vi "CheckShotSuccess.vi"(6 "Vertical Edges":T2(array[cluster]) {"Point2 (Real-World)"."Y" format="%.2f"; "Point2 (Real-World)"."X" format="%.2f"; "Point1 (Real-World)"."Y" format="%.2f"; "Point1 (Real-World)"."X" format="%.2f"; "Point2 (Pixels)"."Y" format="%.2f"; "Point2 (Pixels)"."X" format="%.2f"; "Point1 (Pixels)"."Y" format="%.2f"; "Point1 (Pixels)"."X" format="%.2f"}, 7 "Pixel/mm":dbl format="%#_13g", 8 "error in":errorcluster, 9 "File Path":path, 10 "CameraSettings":T4={"Brightness"=0, "Contrast"=0.0, "Threshold"=50.0}, 11 "Session In":T5) -> (0 "error out":errorcluster, 1 "Image":T1(plugin-control), 2 "Success?":bool, 3 "Session Out":T5, 4 "X distance Out":sgl, 5 "XYPuck":cluster{sgl, sgl})   [LabVIEW 2017]
uses:
  <vilib>/userdefined/High Color/IMAQdx.ctl
panel:
  in  "HomeXY(pixels)":cluster{dbl, dbl}
  out "Vertical Edges[0].Point1 (Pixels).X":sgl
  out "Circles[0].Position.X":sgl
  out "Puck":T3(array[cluster]) {"Position"."Y" format="%.2f"; "Position"."X" format="%.2f"}
  out "Number of Pucks Found":i32
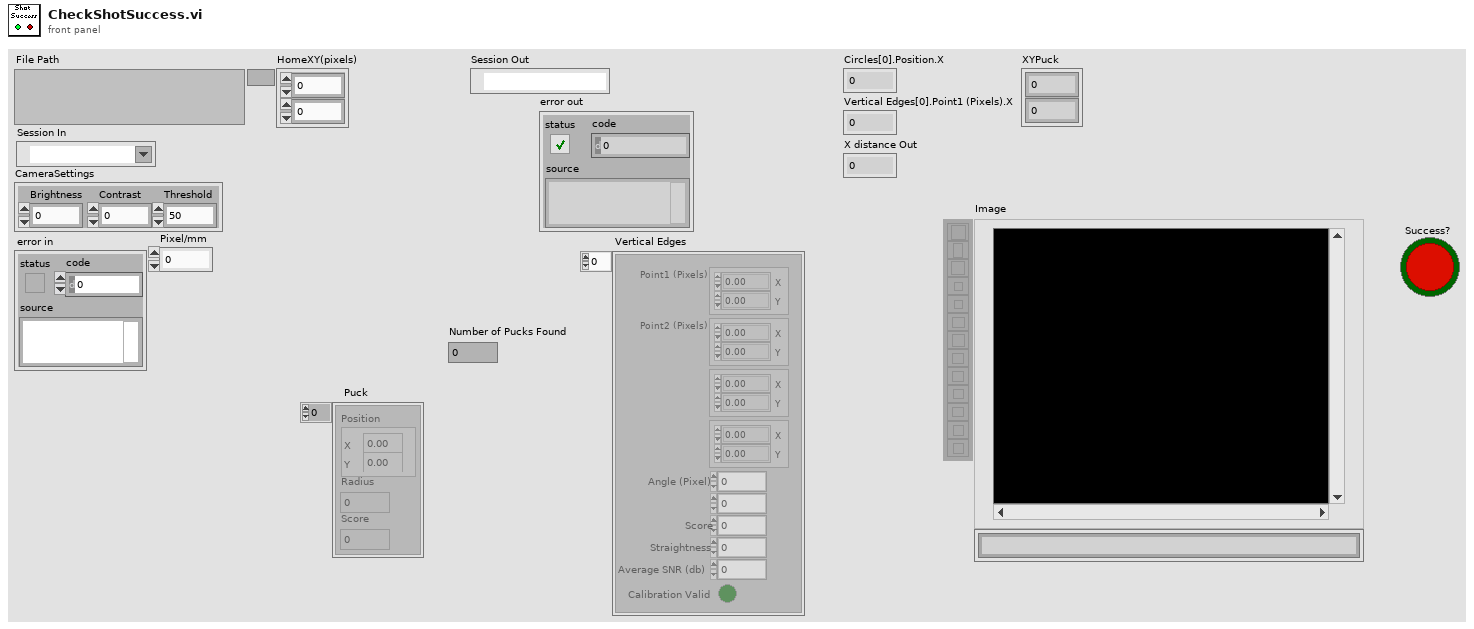
[diagram p1: front panel]
types:
  T1 = typedef "IMAQ Image.ctl" = refnum<image>
  T2 = cluster{"Point1 (Pixels)":cluster{"X":sgl, "Y":sgl}, "Point2 (Pixels)":cluster{"X":sgl, "Y":sgl}, "Point1 (Real-World)":cluster{"X":sgl, "Y":sgl}, "Point2 (Real-World)":cluster{"X":sgl, "Y":sgl}, "Angle (Pixel)":dbl, "Angle (Real-World)":dbl, "Score":dbl, "Straightness":dbl, "Average SNR (db)":dbl, "Calibration Valid":bool}[]
  T3 = cluster{"Position":cluster{"X":sgl, "Y":sgl}, "Radius":dbl, "Score":dbl}[]
  T4 = cluster{"Brightness":i64, "Contrast":dbl, "Threshold":sgl}
  T5 = typedef "IMAQdx.ctl" = refnum<k21>
  T6 = cluster{"Circles[0]":cluster{"Position":cluster{"X":sgl, "Y":sgl}, "Radius":dbl, "Score":dbl}, "Circles[1]":cluster{"Position":cluster{"X":sgl, "Y":sgl}, "Radius":dbl, "Score":dbl}, "Circles[2]":cluster{"Position":cluster{"X":sgl, "Y":sgl}, "Radius":dbl, "Score":dbl}, "Circles[3]":cluster{"Position":cluster{"X":sgl, "Y":sgl}, "Radius":dbl, "Score":dbl}, "Circles[4]":cluster{"Position":cluster{"X":sgl, "Y":sgl}, "Radius":dbl, "Score":dbl}, "Circles[5]":cluster{"Position":cluster{"X":sgl, "Y":sgl}, "Radius":dbl, "Score":dbl}, "Circles[6]":cluster{"Position":cluster{"X":sgl, "Y":sgl}, "Radius":dbl, "Score":dbl}, "Circles[7]":cluster{"Position":cluster{"X":sgl, "Y":sgl}, "Radius":dbl, "Score":dbl}, "Circles[8]":cluster{"Position":cluster{"X":sgl, "Y":sgl}, "Radius":dbl, "Score":dbl}}
  T7 = cluster{"Vertical Edges[0]":cluster{"Point1 (Pixels)":cluster{"X":sgl, "Y":sgl}, "Point2 (Pixels)":cluster{"X":sgl, "Y":sgl}, "Point1 (Real-World)":cluster{"X":sgl, "Y":sgl}, "Point2 (Real-World)":cluster{"X":sgl, "Y":sgl}, "Angle (Pixel)":dbl, "Angle (Real-World)":dbl, "Score":dbl, "Straightness":dbl, "Average SNR (db)":dbl, "Calibration Valid":bool}, "Vertical Edges[1]":cluster{"Point1 (Pixels)":cluster{"X":sgl, "Y":sgl}, "Point2 (Pixels)":cluster{"X":sgl, "Y":sgl}, "Point1 (Real-World)":cluster{"X":sgl, "Y":sgl}, "Point2 (Real-World)":cluster{"X":sgl, "Y":sgl}, "Angle (Pixel)":dbl, "Angle (Real-World)":dbl, "Score":dbl, "Straightness":dbl, "Average SNR (db)":dbl, "Calibration Valid":bool}, "Vertical Edges[2]":cluster{"Point1 (Pixels)":cluster{"X":sgl, "Y":sgl}, "Point2 (Pixels)":cluster{"X":sgl, "Y":sgl}, "Point1 (Real-World)":cluster{"X":sgl, "Y":sgl}, "Point2 (Real-World)":cluster{"X":sgl, "Y":sgl}, "Angle (Pixel)":dbl, "Angle (Real-World)":dbl, "Score":dbl, "Straightness":dbl, "Average SNR (db)":dbl, "Calibration Valid":bool}, "Vertical Edges[3]":cluster{"Point1 (Pixels)":cluster{"X":sgl, "Y":sgl}, "Point2 (Pixels)":cluster{"X":sgl, "Y":sgl}, "Point1 (Real-World)":cluster{"X":sgl, "Y":sgl}, "Point2 (Real-World)":cluster{"X":sgl, "Y":sgl}, "Angle (Pixel)":dbl, "Angle (Real-World)":dbl, "Score":dbl, "Straightness":dbl, "Average SNR (db)":dbl, "Calibration Valid":bool}, "Vertical Edges[4]":cluster{"Point1 (Pixels)":cluster{"X":sgl, "Y":sgl}, "Point2 (Pixels)":cluster{"X":sgl, "Y":sgl}, "Point1 (Real-World)":cluster{"X":sgl, "Y":sgl}, "Point2 (Real-World)":cluster{"X":sgl, "Y":sgl}, "Angle (Pixel)":dbl, "Angle (Real-World)":dbl, "Score":dbl, "Straightness":dbl, "Average SNR (db)":dbl, "Calibration Valid":bool}, "Vertical Edges[5]":cluster{"Point1 (Pixels)":cluster{"X":sgl, "Y":sgl}, "Point2 (Pixels)":cluster{"X":sgl, "Y":sgl}, "Point1 (Real-World)":cluster{"X":sgl, "Y":sgl}, "Point2 (Real-World)":cluster{"X":sgl, "Y":sgl}, "Angle (Pixel)":dbl, "Angle (Real-World)":dbl, "Score":dbl, "Straightness":dbl, "Average SNR (db)":dbl, "Calibration Valid":bool}, "Vertical Edges[6]":cluster{"Point1 (Pixels)":cluster{"X":sgl, "Y":sgl}, "Point2 (Pixels)":cluster{"X":sgl, "Y":sgl}, "Point1 (Real-World)":cluster{"X":sgl, "Y":sgl}, "Point2 (Real-World)":cluster{"X":sgl, "Y":sgl}, "Angle (Pixel)":dbl, "Angle (Real-World)":dbl, "Score":dbl, "Straightness":dbl, "Average SNR (db)":dbl, "Calibration Valid":bool}, "Vertical Edges[7]":cluster{"Point1 (Pixels)":cluster{"X":sgl, "Y":sgl}, "Point2 (Pixels)":cluster{"X":sgl, "Y":sgl}, "Point1 (Real-World)":cluster{"X":sgl, "Y":sgl}, "Point2 (Real-World)":cluster{"X":sgl, "Y":sgl}, "Angle (Pixel)":dbl, "Angle (Real-World)":dbl, "Score":dbl, "Straightness":dbl, "Average SNR (db)":dbl, "Calibration Valid":bool}, "Vertical Edges[8]":cluster{"Point1 (Pixels)":cluster{"X":sgl, "Y":sgl}, "Point2 (Pixels)":cluster{"X":sgl, "Y":sgl}, "Point1 (Real-World)":cluster{"X":sgl, "Y":sgl}, "Point2 (Real-World)":cluster{"X":sgl, "Y":sgl}, "Angle (Pixel)":dbl, "Angle (Real-World)":dbl, "Score":dbl, "Straightness":dbl, "Average SNR (db)":dbl, "Calibration Valid":bool}}
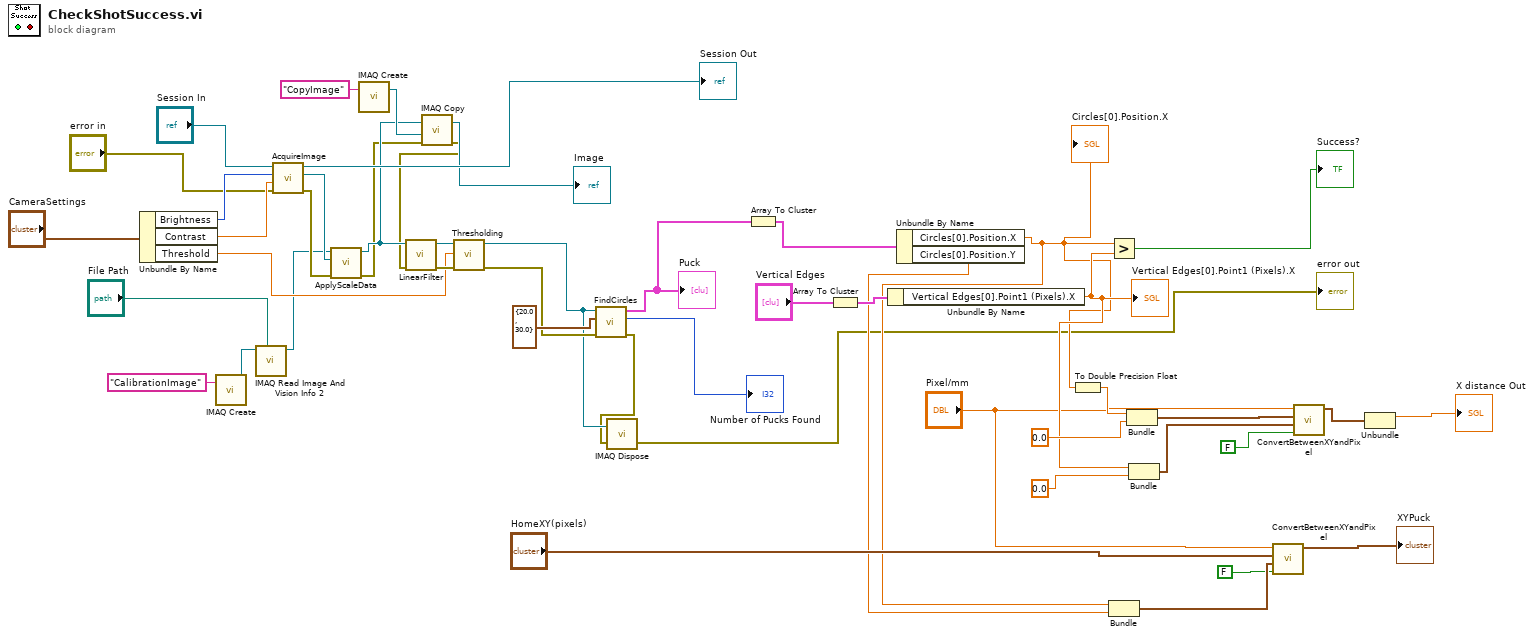
[diagram p0: block diagram]
diagram:
  n1 = Unbundle By Name("CameraSettings") -> ("Brightness"=w38:i64, "Contrast"=w37:dbl, "Threshold"=w35:sgl)
  n2 = call "IMAQ Create"("Image Name"="CalibrationImage") -> ("New Image"=w42:T1)  [unwired: 4 in, 1 out]
  n3 = call "IMAQ Read Image And Vision Info 2"("File Path"="File Path", "Image"=w42) -> ("Image Out"=w34:T1)  [unwired: 7 in, 2 out]
  n4 = call "AcquireImage.vi"("error in"="error in", "Contrast"=w37, "Brightness"=w38, "Session In"="Session In") -> ("error out"=w47:errorcluster, "Image"=w45:T1, "Session Out"=→"Session Out":T5)  [unwired: 4 in]
  n5 = call "ApplyScaleData.vi"("error in (no error)"=w47, "ImageIn"=w45, "CalibImage"=w34) -> ("error out"=w5:errorcluster, "Corrected Image"=w7:T1)  [unwired: 7 in]
  n6 = call "IMAQ Create"("Image Name"="CopyImage") -> ("New Image"=w8:T1)  [unwired: 4 in, 1 out]
  n7 = call "IMAQ Copy"("error in (no error)"=w5, "Image Dst"=w8, "Image Src"=w7) -> ("error out"=w4:errorcluster, "Image Dst Out"=→"Image":T1)  [unwired: 3 in]
  n8 = call "LinearFilter.vi"("error in (no error)"=w4, "Image Src"=w7) -> ("error out"=w46:errorcluster, "Image"=w48:T1)  [unwired: 8 in]
  n9 = call "Thresholding.vi"("error in (no error)"=w46, "Threshold Value"=w35, "Image Src"=w48) -> ("error out"=w26:errorcluster, "Image"=w3:T1)  [unwired: 7 in]
  n10 = call "FindCircles.vi"("error in (no error)"=w26, "Circle Descriptor"=cluster{"Max Radius":dbl, "Min Radius":dbl} {"Max Radius"=20.0, "Min Radius"=30.0}, "Image"=w3) -> ("error out"=w2:errorcluster, "Number of Matches Returned"=→"Number of Pucks Found":i32, "Circles"=w29:T3)  [unwired: 6 in]
  "Puck" <- w29
  n11 = call "IMAQ Dispose"("Image"=w3, "error in (no error)"=w2) -> ("error out"=→"error out":errorcluster)  [unwired: 4 in]
  n12 = Array To Cluster(array=w29) -> (cluster=w28:T6)
  n13 = Array To Cluster(array="Vertical Edges") -> (cluster=w30:T7)
  n14 = Unbundle By Name(w30) -> ("Vertical Edges[0].Point1 (Pixels).X"=w21:sgl)
  "Vertical Edges[0].Point1 (Pixels).X" <- w21
  n15 = Unbundle By Name(w28) -> ("Circles[0].Position.X"=w14:sgl, "Circles[0].Position.Y"=w13:sgl)
  "Circles[0].Position.X" <- w14
  n16 = To Double Precision Float(number=w14) -> (double precision float=w23:dbl)
  n17 = Greater?(x=w14, y=w21) -> (0:→"Success?":bool)
  n18 = Bundle("X"=w14, "Y"=w13) -> (w12:cluster{"X":sgl, "Y":sgl})  [unwired: 1 in]
  n19 = Bundle(w23, 0.0) -> (w22:cluster{dbl, dbl})  [unwired: 1 in]
  n20 = Bundle("X"=w21, sgl 0.0) -> (w20:cluster{"X":sgl, sgl})  [unwired: 1 in]
  n21 = call "ConvertBetweenXYandPixel.vi"("XYtoPixels"=FALSE, "PointToConvert"=w12, "HomeXY(pixels)"="HomeXY(pixels)", "Pixel/mm"="Pixel/mm") -> ("Point"=→"XYPuck":cluster{sgl, sgl})  [unwired: 7 in]
  n22 = call "ConvertBetweenXYandPixel.vi"("XYtoPixels"=FALSE, "PointToConvert"=w20, "HomeXY(pixels)"=w22, "Pixel/mm"="Pixel/mm") -> ("Point"=w18:cluster{sgl, sgl})  [unwired: 7 in]
  n23 = Unbundle(w18) -> (→"X distance Out":sgl)  [unwired: 1 out]
